vi "Hexadecimal to Image.vi"(8 "error in (no error)":errorcluster, 10 "New Image Path":path, 11 "Hexadecimal Text":string) -> (0 "error out":errorcluster)   [LabVIEW 2013]
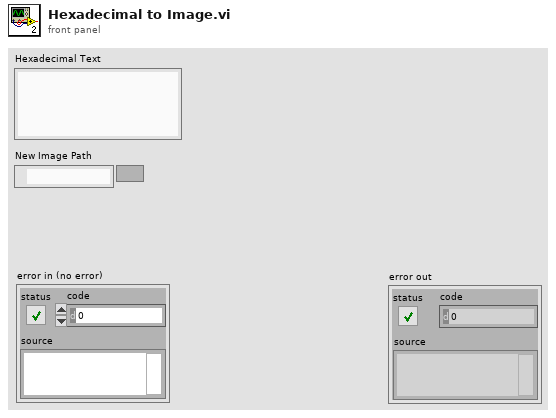
[diagram p1: front panel]
types:
  T1 = enum16{"open", "replace", "create", "open or create", "replace or create", "replace or create with confirmation"}
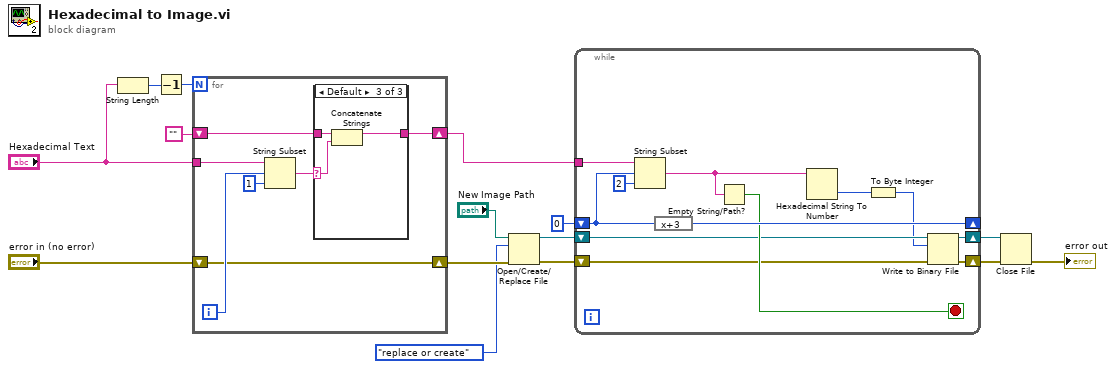
[diagram p0: block diagram]
diagram:
  n1 = String Length(string="Hexadecimal Text") -> (length=w13:i32)
  n2 = Decrement(x=w13) -> (x-1=w12:i32)
  n3 = for {
    N: w12 -> [_]
    tunnel: "Hexadecimal Text" -> [w22]
    shift-right: [w17] -> w10
    shift-left: "" -> [w18]
    shift-right: [w16] -> w8
    shift-left: "error in (no error)" -> [w16]
    i -> [w21]
    n4 = String Subset(string=w22, offset (0)=w21, length (rest)=1 ("length (rest)")) -> (substring=w19:string)
    n5 = case shown="Default" w19 {
      selector: w19 -> [_ _ w27]
      tunnel: w18 -> [w23 w24 w26]
      tunnel: [w23 w24 w25] -> w17
      frame "\r" {
      }
      frame "\n" {
      }
      frame Default {
        n6 = Concatenate Strings(w26, w27) -> (w25:string)
      }
    }
  }
  n7 = Open/Create/Replace File(file path (use dialog)="New Image Path", error in=w8, operation (0:open)=T1."replace or create") -> (refnum out=w6:refnum<file>, error out=w7:errorcluster)  [unwired: 3 in, 1 out]
  n8 = while {
    tunnel: w10 -> [w39]
    shift-right: [w36] -> _
    shift-left: 0 -> [w37]
    shift-right: [w29] -> w5
    shift-left: w7 -> [w32]
    shift-right: [w30] -> w4
    shift-left: w6 -> [w31]
    stop <- w35 stop-if-true
    n9 = String Subset(string=w39, offset (0)=w37, length (rest)=2 ("length (rest)")) -> (substring=w34:string)
    n10 = expression code="x+3"(w37) -> (w36:i32)
    n11 = Empty String/Path?(string/path=w34) -> (empty?=w35:bool)
    n12 = Hexadecimal String To Number(string=w34) -> (number=w33:u32)  [unwired: 2 in, 1 out]
    n13 = To Byte Integer(number=w33) -> (8bit integer=w28:i8)
    n14 = Write to Binary File(file (use dialog)=w31, data=w28, error in=w32) -> (refnum out=w30:refnum<file>, error out=w29:errorcluster)  [unwired: 3 in, 1 out]
  }
  n15 = Close File(refnum=w4, error in=w5) -> (error out=→"error out":errorcluster)  [unwired: 1 out]
